vi "ITC 503 -- upload sweep table.vi"(8 "error in":errorcluster, 9 "Start set point":dbl, 10 "Sweep Table":dbl[][](array[numeric])=[[150.0, 1399.0, 0.0], [20.0, 1399.0, 0.0], [150.0, 1399.0, 0.0], [300.0, 1399.0, 0.0], [295.0, 10.0, 1399.0], [295.0, 10.0, 1399.0]], 11 "ITC503 Address":refnum<visa-resource-name>="GPIB0::24::INSTR") -> (0 "error out":errorcluster, 3 "ITC503 Address OUT":refnum<visa-resource-name>="GPIB0::24::INSTR")   [LabVIEW 2015]
uses:
  Q - not nan -- real.vi
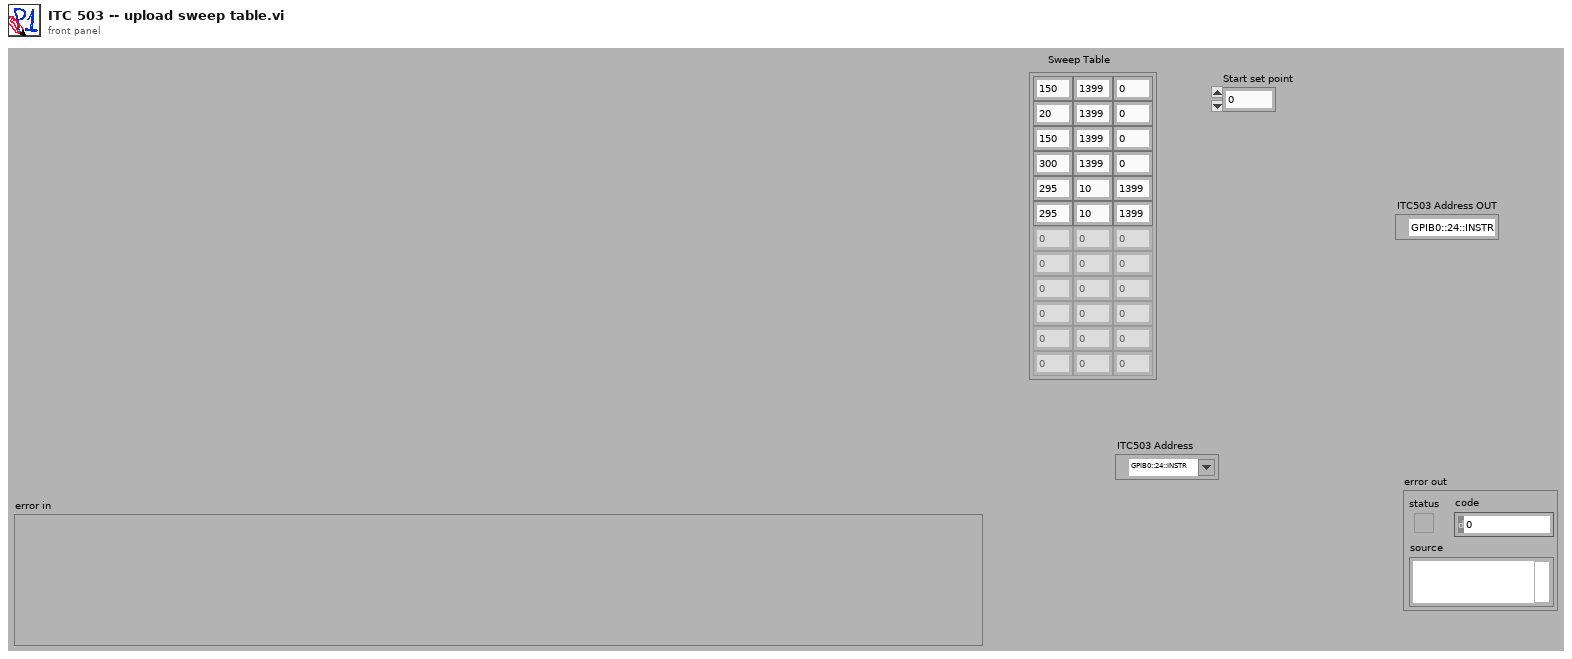
[diagram p1: front panel]
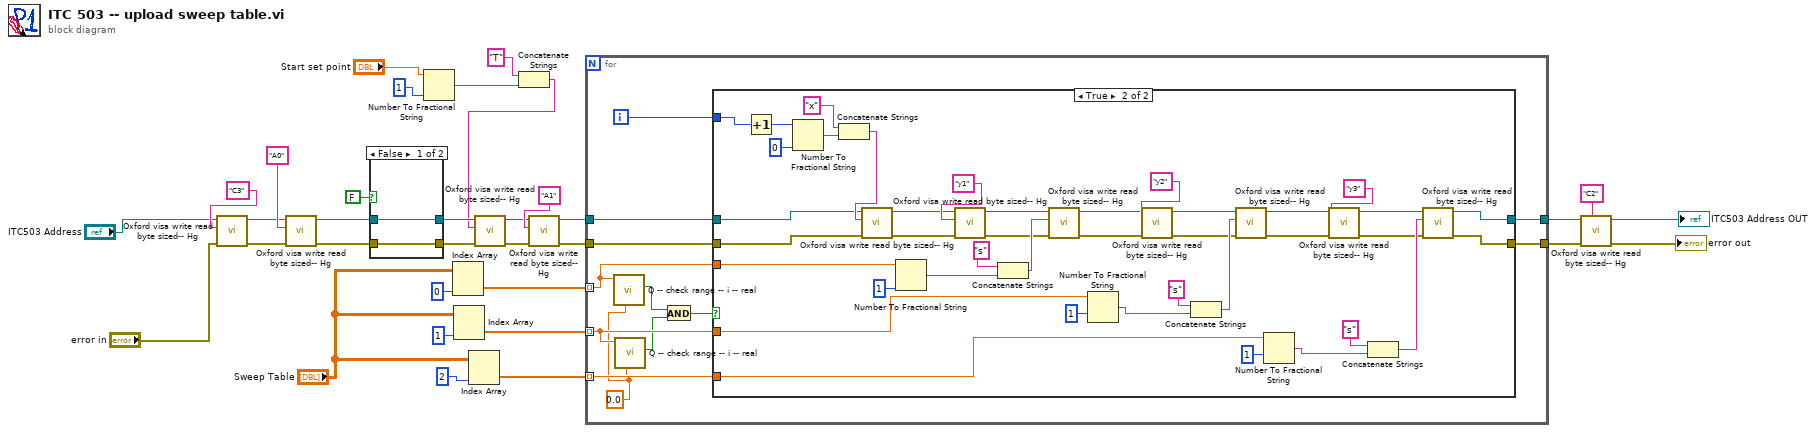
[diagram p0: block diagram]
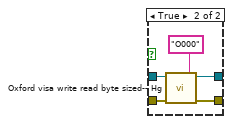
[diagram p2: hidden frame]
diagram:
  n1 = call "Oxford visa write read byte sized-- Hg.vi"("error in (no error)"="error in", "write buffer"="C3" ("Command"), "VISA resource name"="ITC503 Address") -> ("error out"=w27:errorcluster, "VISA resource name out"=w7:refnum<visa-resource-name>)  [unwired: 6 in, 1 out]
  n2 = call "Oxford visa write read byte sized-- Hg.vi"("error in (no error)"=w27, "write buffer"="A0" ("Command"), "VISA resource name"=w7) -> ("error out"=w28:errorcluster, "VISA resource name out"=w8:refnum<visa-resource-name>)  [unwired: 6 in, 1 out]
  n3 = case shown="False" FALSE {
    tunnel: w28 -> [w34 w40]
    tunnel: [w34 w39] -> w25
    tunnel: [w35 w37] -> w9
    tunnel: w8 -> [w35 w36]
    frame False {
    }
    frame True {
      n4 = call "Oxford visa write read byte sized-- Hg.vi"("error in (no error)"=w40, "write buffer"="O000" ("Command"), "VISA resource name"=w36) -> ("error out"=w39:errorcluster, "VISA resource name out"=w37:refnum<visa-resource-name>)  [unwired: 6 in, 1 out]
    }
  }
  n5 = Number To Fractional String(number="Start set point", precision (6)=i16 1) -> (F-format string=w3:string)  [unwired: 2 in]
  n6 = Index Array(array="Sweep Table", index (col)=0 ("disabled index (col)")) -> (element=w15:dbl[])  [unwired: 1 in]
  n7 = Index Array(array="Sweep Table", index (col)=1 ("disabled index (col)")) -> (element=w16:dbl[])  [unwired: 1 in]
  n8 = Index Array(array="Sweep Table", index (col)=2 ("disabled index (col)")) -> (element=w17:dbl[])  [unwired: 1 in]
  n9 = Concatenate Strings("T" ("Command"), w3) -> (w2:string)
  n10 = call "Oxford visa write read byte sized-- Hg.vi"("error in (no error)"=w25, "write buffer"=w2, "VISA resource name"=w9) -> ("error out"=w30:errorcluster, "VISA resource name out"=w10:refnum<visa-resource-name>)  [unwired: 6 in, 1 out]
  n11 = call "Oxford visa write read byte sized-- Hg.vi"("error in (no error)"=w30, "write buffer"="A1" ("Command"), "VISA resource name"=w10) -> ("error out"=w20:errorcluster, "VISA resource name out"=w11:refnum<visa-resource-name>)  [unwired: 6 in, 1 out]
  n12 = for {
    tunnel: w20 -> [w52]
    tunnel: [w49] -> w14
    tunnel: w17 -> [w46] mode=indexing
    tunnel: w16 -> [w45] mode=indexing
    tunnel: w15 -> [w47] mode=indexing
    tunnel: [w50] -> w13
    tunnel: w11 -> [w48]
    i -> [w51]
    w41 = 0.0
    n13 = call "Q -- check range -- i -- real.vi"("lower"=w41, "number"=w47) -> ("in range?"=w44:bool)  [unwired: 7 in, 2 out]
    n14 = call "Q -- check range -- i -- real.vi"("lower"=w41, "number"=w45) -> ("in range?"=w43:bool)  [unwired: 7 in, 2 out]
    n15 = And(x=w44, y=w43) -> (x .and. y?=w42:bool)
    n16 = case shown="True" w42 {
      tunnel: w52 -> [w53 w68]
      tunnel: w51 -> [_ w67]
      tunnel: [w54 w63] -> w50
      tunnel: [w53 w62] -> w49
      tunnel: w48 -> [w54 w58]
      tunnel: w47 -> [_ w57]
      tunnel: w46 -> [_ w56]
      tunnel: w45 -> [_ w55]
      frame False {
      }
      frame True {
        n17 = Increment(x=w67) -> (x+1=w94:i32)
        n18 = Number To Fractional String(number=w94, precision (6)=i16 0) -> (F-format string=w91:string)  [unwired: 2 in]
        n19 = Concatenate Strings("x" ("string"), w91) -> (w90:string)
        n20 = call "Oxford visa write read byte sized-- Hg.vi"("error in (no error)"=w68, "write buffer"=w90, "VISA resource name"=w58) -> ("error out"=w77:errorcluster, "VISA resource name out"=w59:refnum<visa-resource-name>)  [unwired: 6 in, 1 out]
        n21 = Number To Fractional String(number=w57, precision (6)=i16 1) -> (F-format string=w71:string)  [unwired: 2 in]
        n22 = call "Oxford visa write read byte sized-- Hg.vi"("error in (no error)"=w77, "write buffer"="y1" ("string"), "VISA resource name"=w59) -> ("error out"=w76:errorcluster, "VISA resource name out"=w60:refnum<visa-resource-name>)  [unwired: 6 in, 1 out]
        n23 = Concatenate Strings("s" ("string"), w71) -> (w86:string)
        n24 = call "Oxford visa write read byte sized-- Hg.vi"("error in (no error)"=w76, "write buffer"=w86, "VISA resource name"=w60) -> ("error out"=w75:errorcluster, "VISA resource name out"=w61:refnum<visa-resource-name>)  [unwired: 6 in, 1 out]
        n25 = Number To Fractional String(number=w55, precision (6)=i16 1) -> (F-format string=w70:string)  [unwired: 2 in]
        n26 = call "Oxford visa write read byte sized-- Hg.vi"("error in (no error)"=w75, "write buffer"="y2" ("string"), "VISA resource name"=w61) -> ("error out"=w74:errorcluster, "VISA resource name out"=w66:refnum<visa-resource-name>)  [unwired: 6 in, 1 out]
        n27 = Concatenate Strings("s" ("string"), w70) -> (w83:string)
        n28 = call "Oxford visa write read byte sized-- Hg.vi"("error in (no error)"=w74, "write buffer"=w83, "VISA resource name"=w66) -> ("error out"=w73:errorcluster, "VISA resource name out"=w65:refnum<visa-resource-name>)  [unwired: 6 in, 1 out]
        n29 = Number To Fractional String(number=w56, precision (6)=i16 1) -> (F-format string=w69:string)  [unwired: 2 in]
        n30 = call "Oxford visa write read byte sized-- Hg.vi"("error in (no error)"=w73, "write buffer"="y3" ("string"), "VISA resource name"=w65) -> ("error out"=w72:errorcluster, "VISA resource name out"=w64:refnum<visa-resource-name>)  [unwired: 6 in, 1 out]
        n31 = Concatenate Strings("s" ("string"), w69) -> (w78:string)
        n32 = call "Oxford visa write read byte sized-- Hg.vi"("error in (no error)"=w72, "write buffer"=w78, "VISA resource name"=w64) -> ("error out"=w62:errorcluster, "VISA resource name out"=w63:refnum<visa-resource-name>)  [unwired: 6 in, 1 out]
      }
    }
  }
  n33 = call "Oxford visa write read byte sized-- Hg.vi"("error in (no error)"=w14, "write buffer"="C2" ("Command"), "VISA resource name"=w13) -> ("error out"=→"error out":errorcluster, "VISA resource name out"=→"ITC503 Address OUT":refnum<visa-resource-name>)  [unwired: 6 in, 1 out]
